vi "setSetpoint.vi"(8 "error in (no error)":errorcluster, 9 "Force Setpoint":dbl[unit], 10 "ILC in":refnum<class "ILC.lvclass">, 11 "SingleCylinderActuator in":refnum<class "PressureServoCylinderActuator.lvclass">) -> (0 "error out":errorcluster, 2 "ILC out":refnum<class "ILC.lvclass">, 3 "SingleCylinderActuator out":refnum<class "PressureServoCylinderActuator.lvclass">)   [LabVIEW 2015, in "PressureServoCylinderActuator.lvclass"]
uses:
  PressureServoCylinderActuator.lvclass
  <userlib>/Common/ILC/ILC/ILC.lvclass
  PressureServoCylinderActuator.lvclass/PressureServoCylinderActuator.ctl
  IActuatorCylinder/IActuatorCylinder.lvclass
  Calculators/ForceToPressureServoVoltage/ForceToPressureServoVoltage.lvclass
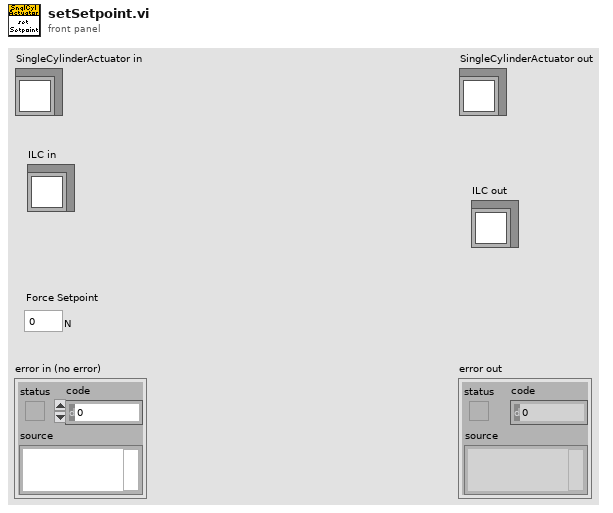
[diagram p1: front panel]
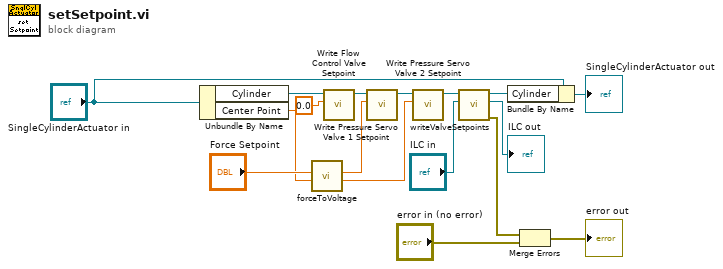
[diagram p0: block diagram]
diagram:
  n1 = Unbundle By Name("SingleCylinderActuator in") -> ("Cylinder"=w10:refnum<class "IActuatorCylinder.lvclass">, "Center Point"=w6:dbl[unit])
  n2 = call "forceToVoltage.vi"("Center Point"=w6, "Force"="Force Setpoint") -> ("Voltage 2"=w4:dbl[unit], "Voltage 1"=w5:dbl[unit])  [unwired: 6 in, 2 out]
  n3 = call-dynamic "Write Flow Control Valve Setpoint.vi"("Flow Control Valve Setpoint"=dbl[unit] 0.0, "IActuatorCylinder in"=w10) -> ("IActuatorCylinder out"=w9:refnum<class "IActuatorCylinder.lvclass">)  [unwired: 9 in]
  n4 = call-dynamic "Write Pressure Servo Valve 1 Setpoint.vi"("Pressure Servo Valve 1 Setpoint"=w5, "IActuatorCylinder in"=w9) -> ("IActuatorCylinder out"=w8:refnum<class "IActuatorCylinder.lvclass">)  [unwired: 9 in]
  n5 = call-dynamic "Write Pressure Servo Valve 2 Setpoint.vi"("Pressure Servo Valve 2 Setpoint"=w4, "IActuatorCylinder in"=w8) -> ("IActuatorCylinder out"=w11:refnum<class "IActuatorCylinder.lvclass">)  [unwired: 9 in]
  n6 = call-dynamic "writeValveSetpoints.vi"("ILC in"="ILC in", "IActuatorCylinder in"=w11) -> ("error out"=w15:errorcluster, "ILC out"=→"ILC out":refnum<class "ILC.lvclass">, "IActuatorCylinder out"=w12:refnum<class "IActuatorCylinder.lvclass">)  [unwired: 7 in]
  n7 = Bundle By Name(cluster="SingleCylinderActuator in", "Cylinder"=w12) -> (→"SingleCylinderActuator out":refnum<class "PressureServoCylinderActuator.lvclass">)
  n8 = Merge Errors(w15, "error in (no error)") -> (→"error out":errorcluster)
